vi "设定输出脉冲个数.vi"(4 "错误输入":errorcluster caption="错误输入（无错误）", 5 "脉冲个数":u32, 6 "通道号":i32, 7 "设备句柄入":i32) -> (0 "错误输出":errorcluster, 3 "设备句柄":i32=1)   [LabVIEW 2016]
uses:
  dll/em9636.dll
panel:
  in  "超时毫秒":i32=1000
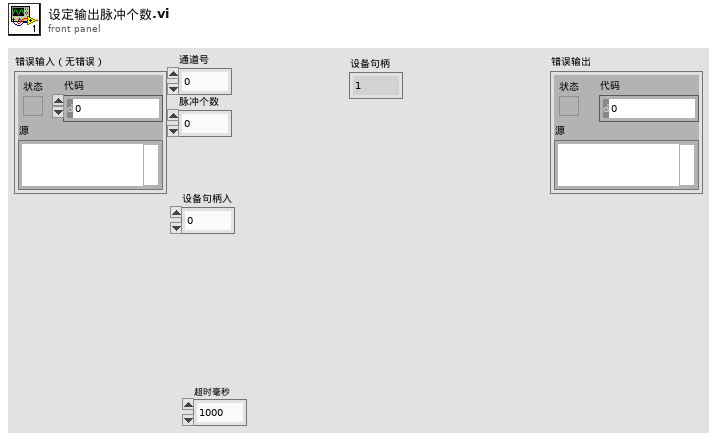
[diagram p1: front panel]
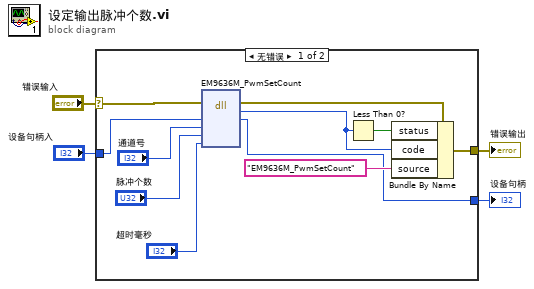
[diagram p0: block diagram]
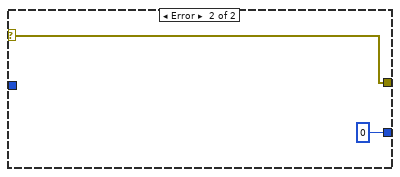
[diagram p2: hidden frame]
diagram:
  n1 = case shown="无错误" "错误输入" {
    selector: "错误输入" -> [w15 w17]
    tunnel: [w11 w17] -> w3
    tunnel: [w7 0 ("错误")] -> w2
    tunnel: "设备句柄入" -> [w9 _]
    frame No Error {
      n2 = dll-call lib="PTH2|abs CUsers\nAdministratorDesktopEM9636original - 副本*EM9636系列_demo_labview(调用DLL方式)dll\nem9636.dll" fn="EM9636M_PwmSetCount"(error in=w15, "设备句柄"=w9, "通道号"="通道号", "脉冲个数"="脉冲个数", "超时毫秒"="超时毫秒") -> (error out=w13:errorcluster, "错误"=w10:i32, "设备句柄"=w7:i32)  [unwired: 5 in, 1 out]
      n3 = Less Than 0?(x=w10) -> (x < 0?=w12:bool)
      n4 = Bundle By Name(cluster=w13, "status"=w12, "code"=w10, "source"="EM9636M_PwmSetCount") -> (w11:errorcluster)
    }
    frame Error {
    }
  }
  "错误输出" <- w3
  "设备句柄" <- w2
